vi "externalAqcuisitionRun.vi"(8 "error in (no error)":errorcluster) -> (0 "error out":errorcluster)   [LabVIEW 2017, in "externalAquisition.lvlib"]
doc: "This is the external Aquisition Main VI. This is responsible for performing all hardware based DAQ, which currently includes handle force data and robot joint encoder data."
uses:
  externalAquisition.lvlib
  UEFGV/Type Def/UEFGV_States.ctl
  internalQueue/TypeDefs/QueueCommands.ctl
  TypeDefs/LoopStates.ctl
  ErrorMonitor/ErrorMonitor.lvlib
  loggingModule/loggingModule.lvlib
  <vilib>/myRIO/Express VI/Onboard IO/I2C/I2C Express VI.xnode
  <vilib>/myRIO/Instrument Drivers/Onboard IO/I2C/vis/Configure.vi
  <vilib>/myRIO/Instrument Drivers/Onboard IO/I2C/I2C.lvlib
  <vilib>/myRIO/Instrument Drivers/Onboard IO/I2C/vis/Write Read.vi
  <vilib>/myRIO/Instrument Drivers/Onboard IO/I2C/typedefs/I2C Transfer Rate.ctl
  <vilib>/myRIO/Instrument Drivers/Onboard IO/I2C/typedefs/I2C User Configuration.ctl
  <vilib>/myRIO/Instrument Drivers/Onboard IO/I2C/typedefs/I2C Configuration.ctl
  <vilib>/myRIO/Common/Instrument Driver Framework/myRIO v1.0/I2C/typedefs/I2C Channels Enum.ctl
  <vilib>/myRIO/Common/Instrument Driver Framework/Utilities/typedefs/Generic FPGA Reference.ctl
  <vilib>/myRIO/Common/Instrument Driver Framework/Utilities/typedefs/myRIO v1.0 Reference.ctl
  <vilib>/myRIO/Common/Instrument Driver Framework/Utilities/typedefs/Hardware Version Enum.ctl
  <vilib>/myRIO/Common/Instrument Driver Framework/Utilities/typedefs/myRIO Generic Hardware Reference.ctl
  <vilib>/myRIO/Instrument Drivers/Onboard IO/I2C/typedefs/I2C Reference.ctl
  <vilib>/myRIO/Instrument Drivers/Onboard IO/I2C/vis/myRIO I2C Open.xnode
  <vilib>/myRIO/Common/Instrument Driver Framework/Utilities/vis/Is FPGA Ref Available.vi
  <vilib>/myRIO/Common/Instrument Driver Framework/myRIO v1.0/I2C/vis/myRIO v1.1 Open I2C.vi
  <vilib>/userdefined/High Color/nirio_resource_hc.ctl
  <vilib>/Instr/_visa.llb/VISA Configure Serial Port (Instr).vi
panel:
  out "stop":bool
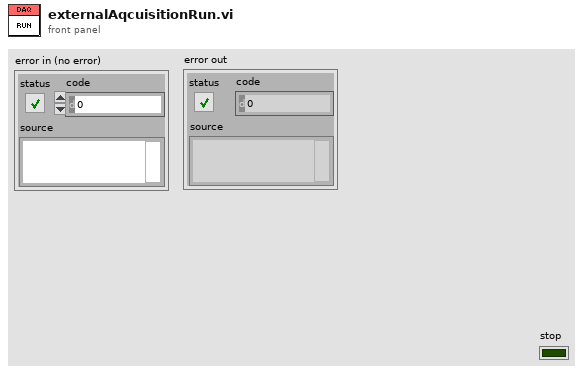
[diagram p1: front panel]
types:
  T1 = typedef "externalAquisition.lvlib/QueueCommands.ctl" = enum16{"get", "set"}
  T2 = typedef "UEFGV_States.ctl" = enum16{"Create", "Get", "Destroy"}
  T3 = typedef "LoopStates.ctl" = enum16{"start", "wait", "run", "end"}
  T4 = typedef "I2C.lvlib/I2C Reference.ctl" = cluster{"myRIO Reference":T5, "I2C Channels Enum":T9, "I2C Configuration":T10}
  T5 = typedef "myRIO Generic Hardware Reference.ctl" = cluster{"myRIO Model":T6, "myRIO Hardware Reference":T7}
  T6 = typedef "Hardware Version Enum.ctl" = enum16{"Unknown", "myRIO-1900", "myRIO-1950", "roboRIO", "NI ELVIS RIO CM"}
  T7 = typedef "myRIO v1.0 Reference.ctl" = cluster{"Generic FPGA Reference":T8, "Allow multiple opens":bool}
  T8 = typedef "Generic FPGA Reference.ctl" = refnum<k20>
  T9 = typedef "I2C Channels Enum.ctl" = enum16{"Not Connected", "A/I2C", "B/I2C", "I2C/I2C"}
  T10 = typedef "I2C.lvlib/I2C Configuration.ctl" = cluster{"I2C Transfer Rate":T11}
  T11 = typedef "I2C.lvlib/I2C Transfer Rate.ctl" = enum16{"Standard mode (100 kbps)", "Fast mode (400 kbps)"}
  T12 = typedef "dataOut.ctl" = cluster{"X0pos":dbl, "Y0pos":dbl, "Z0pos":dbl, "Fx":dbl, "Fy":dbl, "Fz":dbl, "Encoder1":i32, "Encoder2":i32, "Pot1":dbl, "Pot2":dbl, "Theta0":dbl, "Theta1":dbl, "X1pos":dbl, "Y1pos":dbl, "Z1pos":dbl, "X2pos":dbl, "Y2pos":dbl, "Z2pos":dbl, "ErrorOccurred":bool}
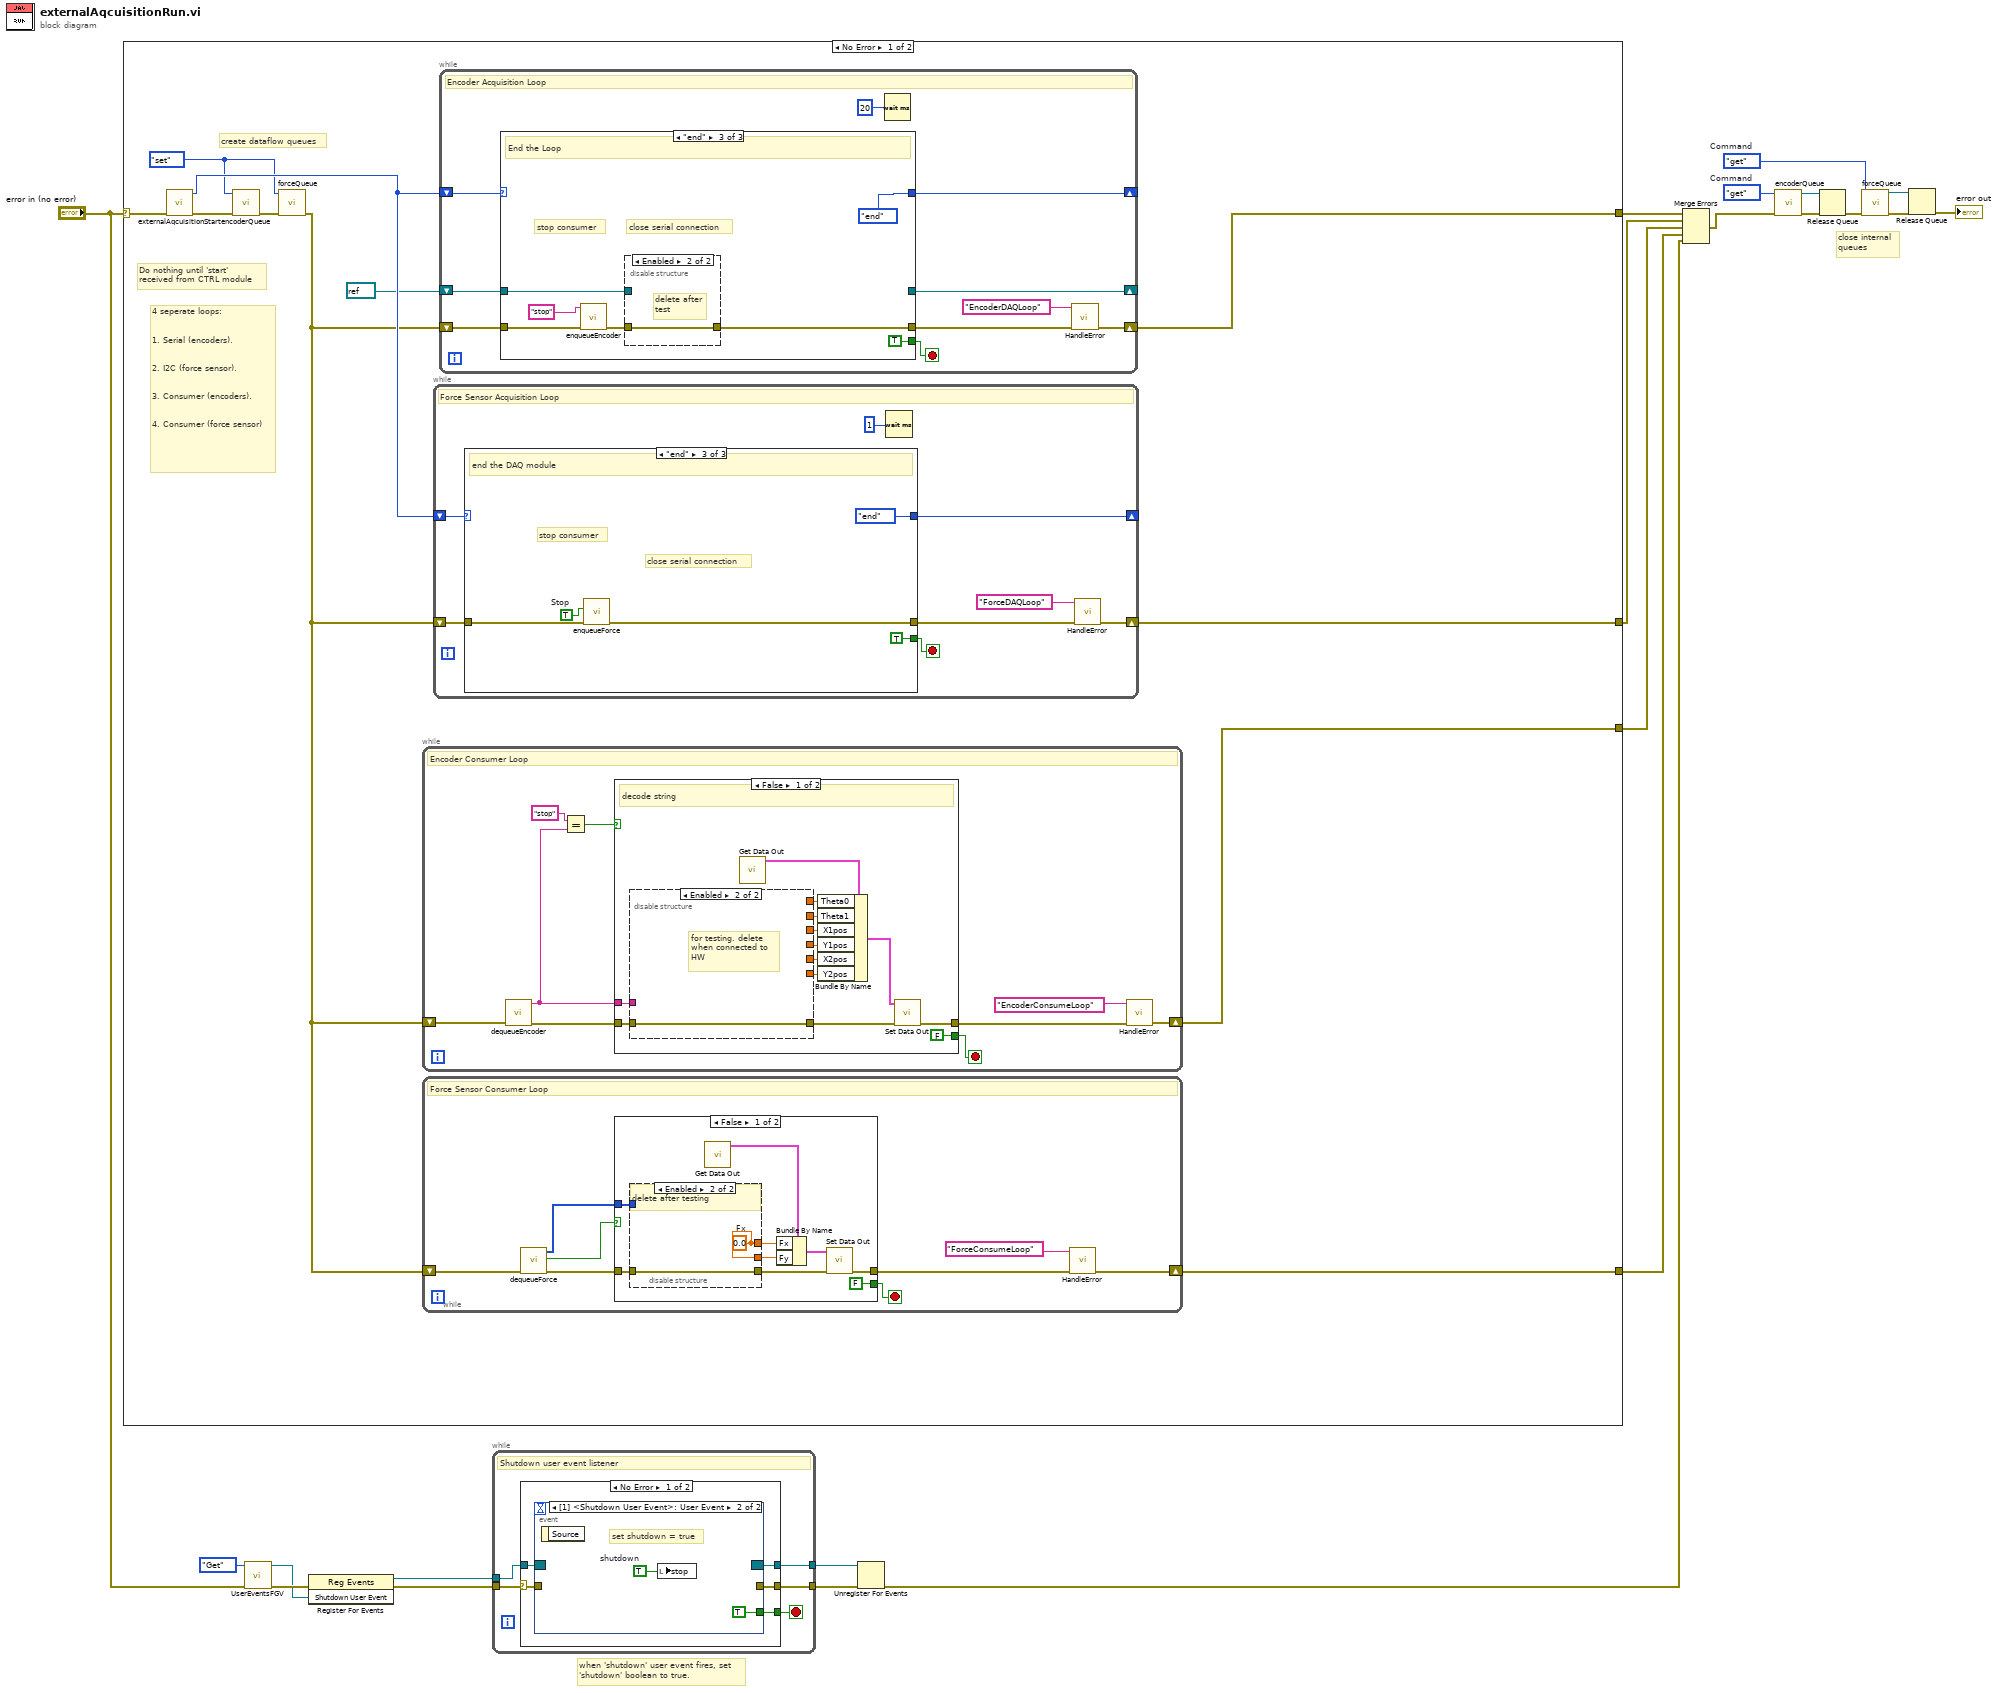
[diagram p0: block diagram]
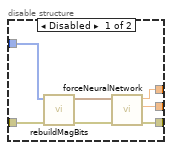
[diagram p2: hidden frame]
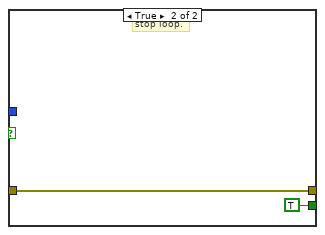
[diagram p3: hidden frame]
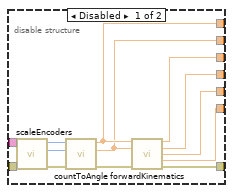
[diagram p4: hidden frame]
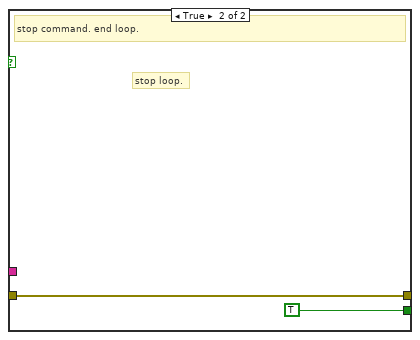
[diagram p5: hidden frame]
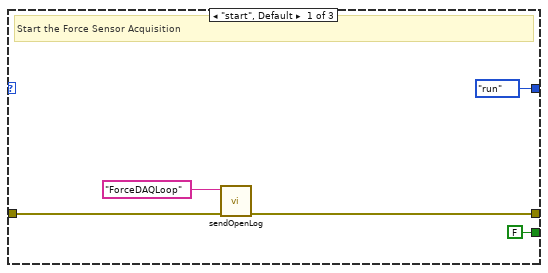
[diagram p6: hidden frame]
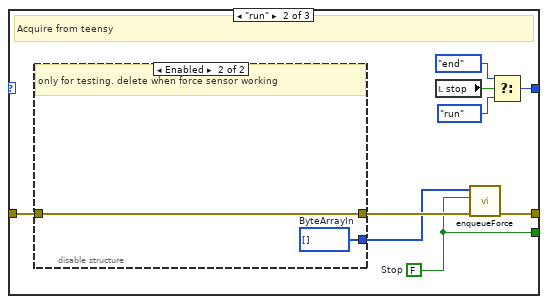
[diagram p7: hidden frame]
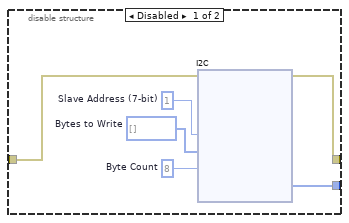
[diagram p8: hidden frame]
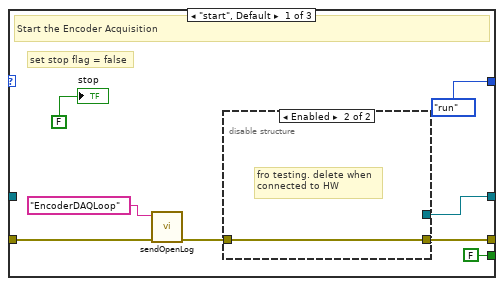
[diagram p9: hidden frame]
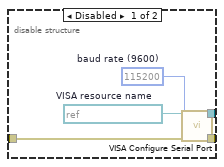
[diagram p10: hidden frame]
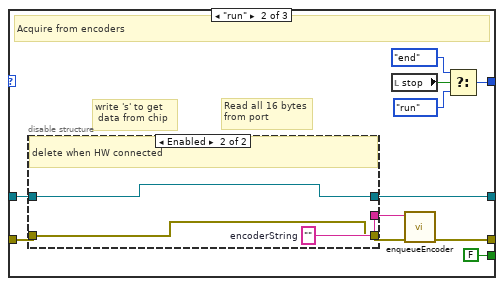
[diagram p11: hidden frame]
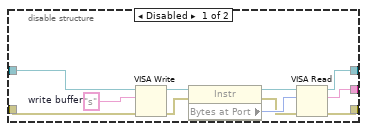
[diagram p12: hidden frame]
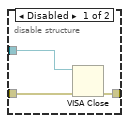
[diagram p13: hidden frame]
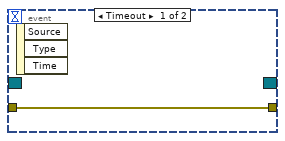
[diagram p15: hidden frame]
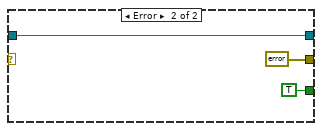
[diagram p16: hidden frame]
diagram:
  w2 = QueueCommands."get"  # Command
  w8 = QueueCommands."get"  # Command
  # "close internal\nqueues"
  # "when 'shutdown' user event fires, set\n'shutdown' boolean to true."
  n1 = case shown="No Error" "error in (no error)" {
    selector: "error in (no error)" -> [w33 w235]
    tunnel: [w26 w235] -> w14
    tunnel: [w23 w235] -> w12
    tunnel: [w24 w235] -> w11
    tunnel: [w25 w235] -> w10
    frame No Error {
      w27 = QueueCommands."set" ("Command")
      # "create dataflow queues"
      # "4 seperate loops:\n\n\n1. Serial (encoders).\n\n\n2. I2C (force sensor).\n\n\n3. Consumer (encoders).\n\n\n4. Consumer (force sensor)"
      # "Do nothing until 'start'\nreceived from CTRL module"
      n2 = call "externalAqcuisitionStart.vi"("error in (no error)"=w33) -> ("error out"=w30:errorcluster, "message out"=w32:T3)  [unwired: 9 in]
      n3 = call "encoderQueue.vi"("error in (no error)"=w30, "Command"=w27) -> ("error out"=w29:errorcluster)  [unwired: 8 in, 1 out]
      n4 = call "forceQueue.vi"("error in (no error)"=w29, "Command"=w27) -> ("error out"=w28:errorcluster)  [unwired: 8 in, 1 out]
      n5 = while {
        shift-right: [w63] -> w24
        shift-left: w28 -> [w70]
        stop <- w66 stop-if-true
        # "Encoder Consumer Loop"
        n6 = call "dequeueEncoder.vi"("error in (no error)"=w70) -> ("error out"=w67:errorcluster, "String"=w62:string)  [unwired: 9 in]
        n7 = Equal?(x="stop", y=w62) -> (x = y?=w68:bool)
        n8 = case shown="False" w68 {
          tunnel: w67 -> [w81 w99]
          tunnel: [w82 w99] -> w64
          tunnel: [FALSE TRUE] -> w66
          tunnel: w62 -> [w71 _]
          frame False {
            # "decode string"
            n9 = disable-structure shown="Enabled" {
              disable-tunnel: w81 -> [w96 w97]
              disable-tunnel: w71 -> [w95 _]
              disable-tunnel: [w90 w97] -> w79
              disable-tunnel: [w89 _] -> w78
              disable-tunnel: [w88 _] -> w77
              disable-tunnel: [w87 _] -> w76
              disable-tunnel: [w86 _] -> w75
              disable-tunnel: [w85 _] -> w74
              disable-tunnel: [w84 _] -> w73
              frame Disabled {
                n10 = call "scaleEncoders.vi"("error in (no error)"=w96, "String"=w95) -> ("error out"=w92:errorcluster, "Encoder1"=w93:u32, "Encoder0"=w94:u32)  [unwired: 7 in]
                n11 = call "countToAngle.vi"("error in (no error)"=w92, "Encoder 1 Count"=w93, "Encoder 0 Count"=w94) -> ("error out"=w91:errorcluster, "Enc 1 angle (rad)"=w88:dbl, "Enc 0 angle (rad)"=w89:dbl)  [unwired: 6 in]
                n12 = call "forwardKinematics.vi"("Theta 0"=w89, "Theta 1"=w88, "error in (no error)"=w91) -> ("Link1X"=w87:dbl, "Link1Y"=w86:dbl, "Link2X"=w85:dbl, "Link2Y"=w84:dbl, "error out"=w90:errorcluster)  [unwired: 8 in]
              }
              frame Enabled {
                # "for testing. delete\nwhen connected to\nHW"
              }
            }
            n13 = call "Get Data Out.vi"() -> ("DataOut"=w72:T12)  [unwired: 10 in, 1 out]
            n14 = Bundle By Name(cluster=w72, "Theta0"=w78, "Theta1"=w77, "X1pos"=w76, "Y1pos"=w75, "X2pos"=w74, "Y2pos"=w73) -> (w80:T12)
            n15 = call "Set Data Out.vi"("error in (no error)"=w79, "DataOut"=w80) -> ("error out"=w82:errorcluster)  [unwired: 9 in]
          }
          frame True {
            # "stop loop."
            # "stop command. end loop."
          }
        }
        n16 = call "HandleError.vi"("error in (no error)"=w64, "Source"="EncoderConsumeLoop") -> ("error out"=w63:errorcluster)  [unwired: 9 in]
      }
      n17 = while {
        shift-right: [w36] -> w23
        shift-left: w28 -> [w41]
        stop <- w39 stop-if-true
        # "Force Sensor Consumer Loop"
        n18 = call "dequeueForce.vi"("error in (no error)"=w41) -> ("error out"=w40:errorcluster, "Stop"=w35:bool, "RawBits"=w34:u8[])  [unwired: 8 in]
        n19 = case shown="False" w35 {
          tunnel: w40 -> [w48 w61]
          tunnel: [w49 w61] -> w37
          tunnel: [FALSE TRUE] -> w39
          tunnel: w34 -> [w47 _]
          frame False {
            n20 = disable-structure shown="Enabled" {
              disable-tunnel: w48 -> [w57 w59]
              disable-tunnel: w47 -> [w56 _]
              disable-tunnel: [w54 w59] -> w46
              disable-tunnel: [w52 w58] -> w43
              disable-tunnel: [w51 w58] -> w42
              frame Disabled {
                n21 = call "rebuildMagBits.vi"("error in (no error)"=w57, "ByteArrayIn"=w56) -> ("error out"=w55:errorcluster, "rawBits"=w53:cluster{u16, u16, u16, u16})  [unwired: 8 in]
                n22 = call "forceNeuralNetwork.vi"("error in (no error)"=w55, "rawBits"=w53) -> ("error out"=w54:errorcluster, "Fy"=w51:dbl, "Fx"=w52:dbl)  [unwired: 7 in]
              }
              frame Enabled {
                w58 = 0.0  # Fx
                # "delete after testing"
              }
            }
            n23 = call "Get Data Out.vi"() -> ("DataOut"=w45:T12)  [unwired: 10 in, 1 out]
            n24 = Bundle By Name(cluster=w45, "Fx"=w43, "Fy"=w42) -> (w44:T12)
            n25 = call "Set Data Out.vi"("error in (no error)"=w46, "DataOut"=w44) -> ("error out"=w49:errorcluster)  [unwired: 9 in]
          }
          frame True {
            # "stop loop."
          }
        }
        n26 = call "HandleError.vi"("error in (no error)"=w37, "Source"="ForceConsumeLoop") -> ("error out"=w36:errorcluster)  [unwired: 9 in]
      }
      n27 = while {
        shift-right: [w106] -> _
        shift-left: w32 -> [w107]
        shift-right: [w100] -> w25
        shift-left: w28 -> [w104]
        stop <- w103 stop-if-true
        # "Force Sensor Acquisition Loop"
        n28 = case shown="\"end\"" w107 {
          tunnel: [LoopStates."run" ("message out") w117 LoopStates."end" ("message out")] -> w106
          tunnel: [w108 w121 w171] -> w101
          tunnel: w104 -> [w110 w116 w172]
          tunnel: [FALSE w114 TRUE] -> w103
          frame "start", Default {
            # "Start the Force Sensor Acquisition"
            n29 = call "sendOpenLog.vi"("error in (no error)"=w110, "source"="ForceDAQLoop" ("Source")) -> ("error out"=w108:errorcluster)  [unwired: 9 in]
          }
          frame "run" {
            w114 = FALSE  # Stop
            # "Acquire from teensy"
            n30 = disable-structure shown="Enabled" {
              disable-tunnel: w116 -> [w127 w169]
              disable-tunnel: [w126 w169] -> w115
              disable-tunnel: [w122 w168] -> w113
              frame Disabled {
                w123 = u32 8  # Byte Count
                w124 = u8[] []  # Bytes to Write
                w125 = u8 1  # Slave Address (7-bit)
                n31 = xnode "I2C"("Slave Address (7-bit)"=w125, "Bytes to Write"=w124, "Byte Count"=w123, "error in (no error)"=w127) -> ("Bytes Read"=w122:u8[], "error out"=w126:errorcluster)
              }
              frame Enabled {
                w168 = u8[] []  # ByteArrayIn
                # "only for testing. delete when force sensor working"
              }
            }
            n32 = local read "stop"() -> (w119:bool)
            n33 = call "enqueueForce.vi"("error in (no error)"=w115, "Stop"=w114, "RawBits"=w113) -> ("error out"=w121:errorcluster)  [unwired: 8 in]
            n34 = Select(t=LoopStates."end" ("message out"), s=w119, f=LoopStates."run" ("message out")) -> (s? t:f=w117:T3)
          }
          frame "end" {
            w170 = TRUE  # Stop
            # "stop consumer"
            # "close serial connection"
            # "end the DAQ module"
            n35 = call "enqueueForce.vi"("error in (no error)"=w172, "Stop"=w170) -> ("error out"=w171:errorcluster)  [unwired: 9 in]
          }
        }
        n36 = Wait (ms)(milliseconds to wait=u32 1) -> ()  [unwired: 1 out]
        n37 = call "HandleError.vi"("error in (no error)"=w101, "Source"="ForceDAQLoop") -> ("error out"=w100:errorcluster)  [unwired: 9 in]
      }
      n38 = while {
        shift-right: [w183] -> _
        shift-left: w32 -> [w184]
        shift-right: [w175] -> w26
        shift-left: w28 -> [w181]
        shift-right: [w179] -> _
        shift-left: refnum<visa-resource-name> refnum ("VISA resource name out") -> [w178]
        stop <- w180 stop-if-true
        # "Encoder Acquisition Loop"
        n39 = case shown="\"end\"" w184 {
          tunnel: [LoopStates."run" ("message out") w200 LoopStates."end" ("message out")] -> w183
          tunnel: [w190 w204 w225] -> w176
          tunnel: w181 -> [w187 w208 w228]
          tunnel: [FALSE FALSE TRUE] -> w180
          tunnel: [w189 w206 _] -> w179
          tunnel: w178 -> [_ w207 w226]
          frame "start", Default {
            # "set stop flag = false"
            # "Start the Encoder Acquisition"
            n40 = call "sendOpenLog.vi"("error in (no error)"=w187, "source"="EncoderDAQLoop" ("Source")) -> ("error out"=w186:errorcluster)  [unwired: 9 in]
            n41 = disable-structure shown="Enabled" {
              disable-tunnel: [w195 w198] -> w190
              disable-tunnel: [w194 _] -> w189
              disable-tunnel: w186 -> [w193 w198]
              frame Disabled {
                w196 = u32 115200  # baud rate (9600)
                w197 = refnum<visa-resource-name> "ASRL2::INSTR"  # VISA resource name
                n42 = call-poly "VISA Configure Serial Port"("VISA resource name"=w197, "baud rate (9600)"=w196, "error in (no error)"=w193) -> ("VISA resource name out"=w194:refnum<visa-resource-name>, "error out"=w195:errorcluster)  [unwired: 11 in]
              }
              frame Enabled {
                # "fro testing. delete when\nconnected to HW"
              }
            }
            "stop" <- FALSE ("stop")
          }
          frame "run" {
            # "Read all 16 bytes\nfrom port"
            # "write 's' to get\n data from chip"
            # "Acquire from encoders"
            n43 = disable-structure shown="Enabled" {
              disable-tunnel: w208 -> [w214 w222]
              disable-tunnel: w207 -> [w213 w221]
              disable-tunnel: [w212 w221] -> w206
              disable-tunnel: [w211 w222] -> w205
              disable-tunnel: [w210 w223] -> w199
              frame Disabled {
                w220 = "s"  # write buffer
                n44 = VISA Write(VISA resource name=w213, write buffer=w220, error in (no error)=w214) -> (VISA resource name out=w219:refnum<visa-resource-name>, error out=w218:errorcluster)  [unwired: 1 out]
                n45 = property class="Instr"(reference=w219, error in=w218) -> (reference out=w216:refnum<visa-resource-name>, error out=w215:errorcluster, "Bytes at Port"=w217:u32)
                n46 = VISA Read(VISA resource name=w216, byte count=w217, error in (no error)=w215) -> (VISA resource name out=w212:refnum<visa-resource-name>, read buffer=w210:string, error out=w211:errorcluster)  [unwired: 1 out]
              }
              frame Enabled {
                w223 = ""  # encoderString
                # "delete when HW connected"
              }
            }
            n47 = local read "stop"() -> (w203:bool)
            n48 = call "enqueueEncoder.vi"("error in (no error)"=w205, "String"=w199) -> ("error out"=w204:errorcluster)  [unwired: 9 in]
            n49 = Select(t=LoopStates."end" ("message out"), s=w203, f=LoopStates."run" ("message out")) -> (s? t:f=w200:T3)
          }
          frame "end" {
            # "close serial connection"
            # "stop consumer"
            # "End the Loop"
            n50 = call "enqueueEncoder.vi"("error in (no error)"=w228, "String"="stop") -> ("error out"=w227:errorcluster)  [unwired: 9 in]
            n51 = disable-structure shown="Enabled" {
              disable-tunnel: w227 -> [w233 w234]
              disable-tunnel: w226 -> [w232 _]
              disable-tunnel: [w231 w234] -> w225
              frame Disabled {
                n52 = VISA Close(VISA resource name=w232, error in (no error)=w233) -> (error out=w231:errorcluster)
              }
              frame Enabled {
                # "delete after\ntest"
              }
            }
          }
        }
        n53 = Wait (ms)(milliseconds to wait=u32 20) -> ()  [unwired: 1 out]
        n54 = call "HandleError.vi"("error in (no error)"=w176, "Source"="EncoderDAQLoop") -> ("error out"=w175:errorcluster)  [unwired: 9 in]
      }
    }
    frame Error {
    }
  }
  n55 = call "UserEventsFGV.vi"("error in (no error)"="error in (no error)", "Command"=UEFGV_States."Get") -> ("error out"=w20:errorcluster, "Shutdown User Event"=w19:refnum<user-event>)  [unwired: 8 in]
  n56 = register-events(error in=w20, w19) -> (reference out=w22:refnum<event-registration>, error out=w17:errorcluster)  [unwired: 1 in]
  n57 = while {
    tunnel: w22 -> [w240]
    tunnel: [w239] -> w21
    tunnel: w17 -> [w237]
    tunnel: [w236] -> w18
    stop <- w238 stop-if-true
    # "Shutdown user event listener"
    n58 = case shown="No Error" w237 {
      selector: w237 -> [w242 _]
      tunnel: w240 -> [w245 w250]
      tunnel: [w244 w250] -> w239
      tunnel: [w243 TRUE] -> w238
      tunnel: [w241 errorcluster {"status"=FALSE, "code"=0, "source"=""} ("error out")] -> w236
      frame No Error {
        n59 = event shown="[1] <Shutdown User Event>: User Event" {
          selector: w245 -> [_ _]
          dyn-events: [_ _] -> w244
          timeout: _ -> [_ _]
          tunnel: w242 -> [w246 _]
          tunnel: [w246 _] -> w241
          tunnel: [_ TRUE] -> w243
          event Timeout {
            n60 = event-data() -> ()  [unwired: 1 in, 3 out]
          }
          event User Event {
            w247 = TRUE  # shutdown
            # "set shutdown = true"
            n61 = event-data() -> ()  [unwired: 1 in, 1 out]
            n62 = local write "stop"(w247) -> ()
          }
        }
      }
      frame Error {
      }
    }
  }
  n63 = Unregister For Events(event registration refnum=w21, error in=w18) -> (error out=w13:errorcluster)
  n64 = Merge Errors(w14, w10, w11, w12, w13) -> (w9:errorcluster)
  n65 = call "encoderQueue.vi"("error in (no error)"=w9, "Command"=w8) -> ("error out"=w6:errorcluster, "queue out"=w7:refnum<queue>)  [unwired: 8 in]
  n66 = Release Queue(queue=w7, error in (no error)=w6) -> (error out=w5:errorcluster)  [unwired: 1 in, 2 out]
  n67 = call "forceQueue.vi"("error in (no error)"=w5, "Command"=w2) -> ("error out"=w4:errorcluster, "queue out"=w3:refnum<queue>)  [unwired: 8 in]
  n68 = Release Queue(queue=w3, error in (no error)=w4) -> (error out=→"error out":errorcluster)  [unwired: 1 in, 2 out]
